vi "getFontFromDocument.vi"(8 "error in (no error)":errorcluster, 11 "xwpfRun in":refnum<class "xwpfRun.lvclass">) -> (0 "error out":errorcluster, 3 "xwpfRun out":refnum<class "xwpfRun.lvclass">)   [LabVIEW 2017, in "Word_Specific.lvlib" / "xwpfRun.lvclass"]
uses:
  xwpfRun.lvclass
  xwpfRun.lvclass/xwpfRun.ctl
  C:/Program Files (x86)/National Instruments/LabVIEW 2017/vi.lib/BenjaminR/LabVIEW NPOI/lib/NPOI 2.1.1/NPOI.OOXML.dll
  Program Files (x86)/National Instruments/LabVIEW 2017/vi.lib/BenjaminR/LabVIEW NPOI/lib/NPOI 2.1.1/NPOI.OOXML.dll
  Styles/Style/Style.lvclass
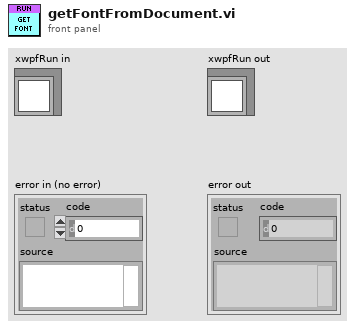
[diagram p1: front panel]
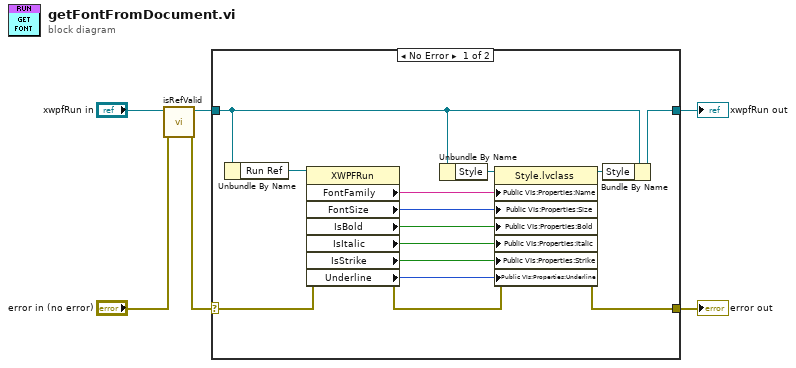
[diagram p0: block diagram]
diagram:
  n1 = call-dynamic "isRefValid.vi"("error in (no error)"="error in (no error)", "xwpfRun in"="xwpfRun in") -> ("error out"=w2:errorcluster, "xwpfRun out"=w3:refnum<class "xwpfRun.lvclass">)  [unwired: 8 in]
  n2 = case shown="No Error" w2 {
    selector: w2 -> [w20 w22]
    tunnel: [w18 w22] -> w6
    tunnel: [w19 w21] -> w4
    tunnel: w3 -> [w17 w21]
    frame No Error {
      n3 = Unbundle By Name(w17) -> ("Run Ref"=w16:refnum<k24>)
      n4 = property class="XWPFRun"(reference=w16, error in=w20) -> (error out=w13:errorcluster, "FontFamily"=w12:string, "FontSize"=w11:i32, "IsBold"=w10:bool, "IsItalic"=w9:bool, "IsStrike"=w8:bool, "Underline"=w7:i32)  [unwired: 1 out]
      n5 = Unbundle By Name(w17) -> ("Style"=w15:refnum<class "Style.lvclass">)
      n6 = property class="Style.lvclass"(reference=w15, error in=w13, "Public VIs:Properties:Name"=w12, "Public VIs:Properties:Size"=w11, "Public VIs:Properties:Bold"=w10, "Public VIs:Properties:Italic"=w9, "Public VIs:Properties:Strike"=w8, "Public VIs:Properties:Underline"=w7) -> (reference out=w14:refnum<class "Style.lvclass">, error out=w18:errorcluster)
      n7 = Bundle By Name(cluster=w17, "Style"=w14) -> (w19:refnum<class "xwpfRun.lvclass">)
    }
    frame Error {
    }
  }
  "error out" <- w6
  "xwpfRun out" <- w4
